vi "grab and max filter.vi"() -> ()   [LabVIEW 2011]
uses:
  <userlib>/labvvis/New Image/New Image (Grey).vi
  <userlib>/labvvis/labvvis.lvlib
panel:
  out "Error":string
  in  "Boolean":bool=TRUE
  in  "Mask":i8[][](array[numeric])=[[-1, -1, 0], [-1, 0, 1], [0, 1, 1]]
  out "new picture":picture
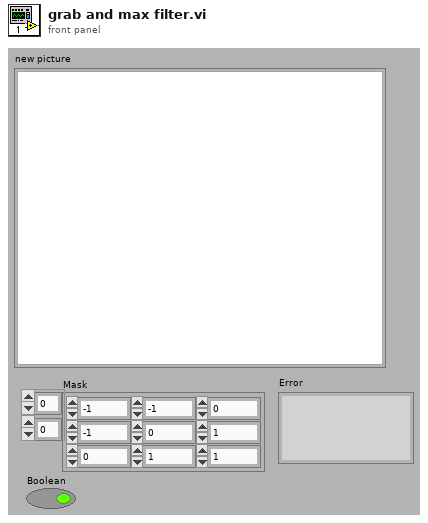
[diagram p1: front panel]
types:
  T1 = typedef "labvvis.lvlib/VVIS Image.ctl" = cluster{"Image ID":i16, "Channel ID":i16}
  T2 = typedef "imagedata.ctl" = cluster{"image type":i32, "image depth":i32, "image":u8[], "mask":u8[], "colors":u32[], "Rectangle":cluster{"left":i16, "top":i16, "right":i16, "bottom":i16}}
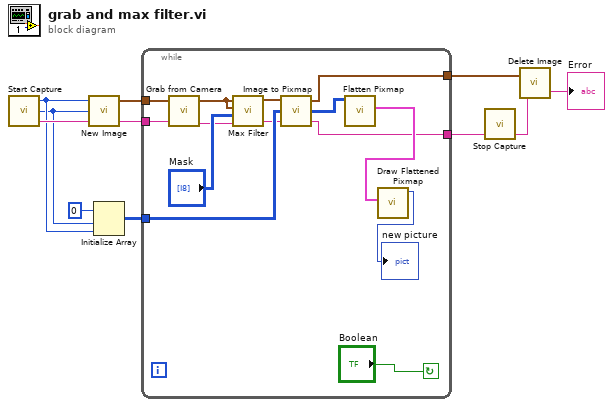
[diagram p0: block diagram]
diagram:
  n1 = call <userlib>:"Start Capture.vi"() -> ("Error"=w6:string, "Height"=w4:i32, "Width"=w5:i32)  [unwired: 3 in]
  n2 = call-poly <userlib>:"New Image.vi"("Error"=w6, "Height"=w4, "Width"=w5) -> ("Error"=w8:string, "VVIS Image"=w9:T1)  [unwired: 1 in]
  n3 = Initialize Array(0, w4, w5) -> (w10:i32[][])
  n4 = while {
    tunnel: w10 -> [w21]
    tunnel: w9 -> [w22]
    tunnel: w8 -> [w15]
    tunnel: [w13] -> w7
    tunnel: [w12] -> w3
    stop <- "Boolean" continue-if-true
    n5 = call <userlib>:"Grab from Camera.vi"("Error"=w15, "Image"=w22) -> ("Error"=w16:string, "Image"=w20:T1)  [unwired: 1 in, 1 out]
    n6 = call <userlib>:"Max Filter.vi"("Error"=w16, "Mask"="Mask", "Output Image"=w20, "Input Image"=w20) -> ("Error"=w17:string, "Input Image"=w18:T1)  [unwired: 1 in, 1 out]
    n7 = call <userlib>:"Image to Pixmap.vi"("Error"=w17, "Output Pixmap"=w21, "Image"=w18) -> ("Error"=w12:string, "Output Pixmap"=w14:u32[][], "Image"=w13:T1)
    n8 = call <vilib>:"Flatten Pixmap.vi"("24-bit pixmap"=w14) -> ("image data"=w24:T2)  [unwired: 10 in]
    n9 = call <vilib>:"Draw Flattened Pixmap.vi"("image data"=w24) -> ("new picture"=→"new picture":picture)  [unwired: 8 in]
  }
  n10 = call <userlib>:"Stop Capture.vi"("Error"=w3) -> ("Error"=w2:string)  [unwired: 4 in]
  n11 = call <userlib>:"Delete Image.vi"("Error"=w2, "Image"=w7) -> ("Error"=→"Error":string)  [unwired: 1 in]
